vi "Untitled 1, Aula 4 (João).vi"() -> (1 "Potencia ativa A":dbl[](graph), 4 "Potencia ativa B":dbl[](graph), 7 "Potencia ativa C":dbl[](graph), 9 "timestamp":dbl[](array[numeric]))   [LabVIEW 2024]
uses:
  <vilib>/numeric/Random Number (Range) DBL.vi
panel:
  out "Tensão fase C":dbl[](array[numeric])
  out "Corrente fase C":dbl[](array[numeric])
  out "Potencia ativa":dbl[](array[numeric])
  out "Fator portencia 3":dbl
  in  "Limite inferior FP 3":dbl
  in  "Limite superior FP 3":dbl=100.0
  out "Corrente fase B":dbl[](array[numeric])
  out "Tensão fase B":dbl[](array[numeric])
  out "Potencia ativa B":dbl[](array[numeric])
  out "Fator portencia 2":dbl
  in  "Limite inferior FP 2":dbl
  in  "Limite superior FP 2":dbl=100.0
  out "Potencia ativa A":dbl[](array[numeric])
  out "Fator portencia":dbl
  out "Corrente fase A":dbl[](array[numeric])
  out "Tensão fase A":dbl[](array[numeric])
  in  "Limite inferior FP":dbl
  in  "Limite superior FP":dbl=100.0
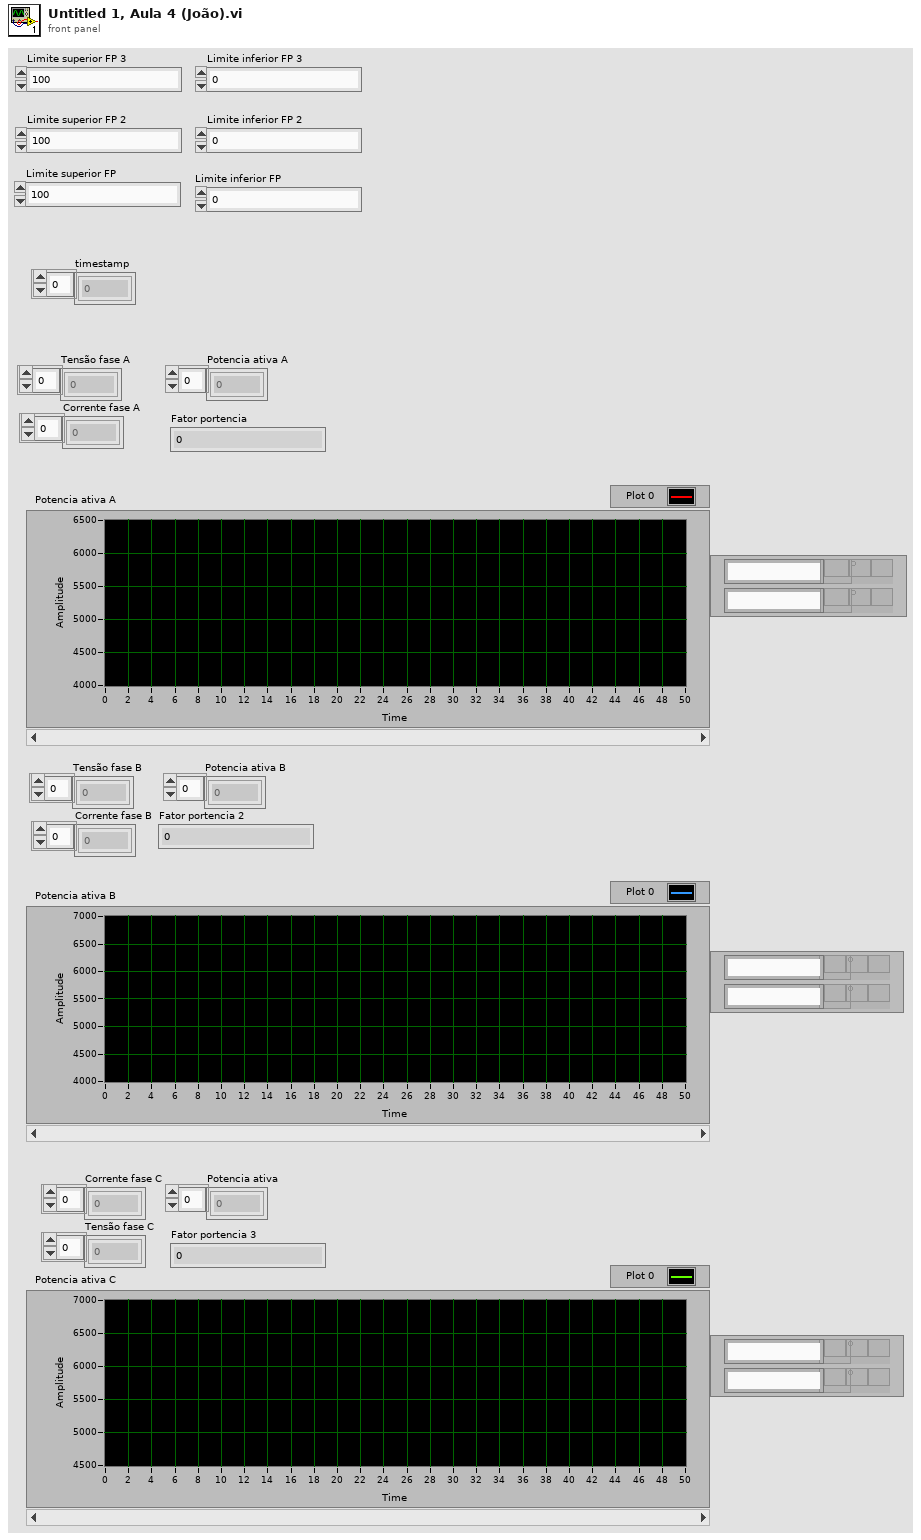
[diagram p1: front panel]
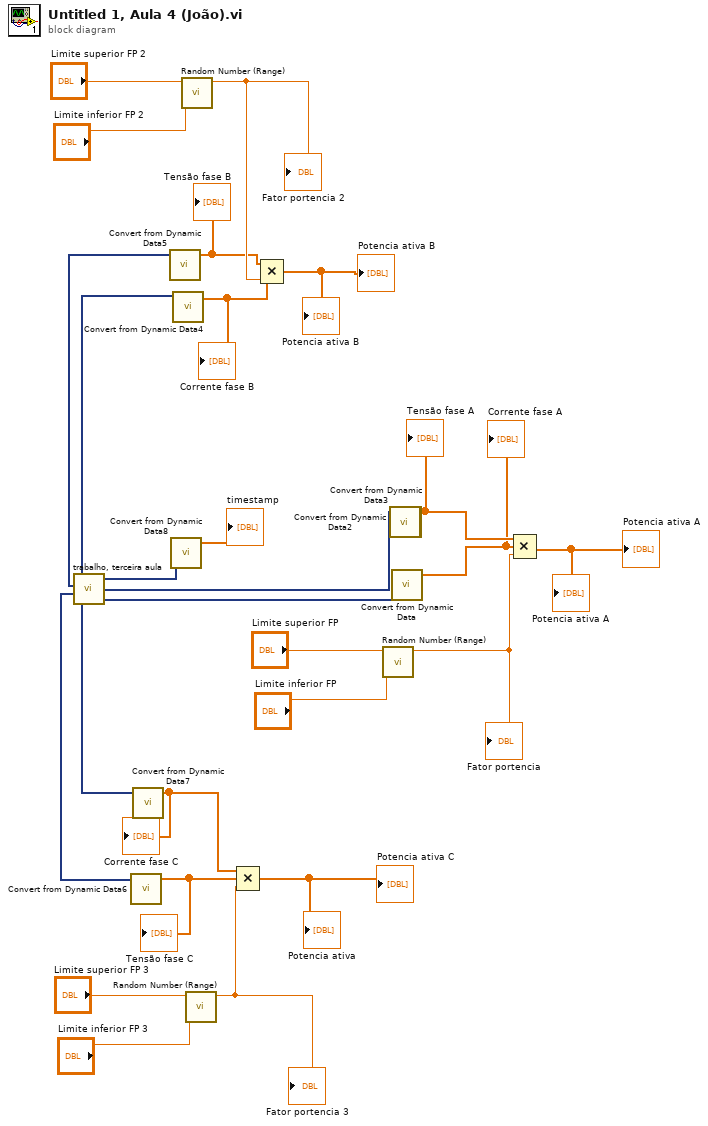
[diagram p0: block diagram]
diagram:
  n1 = call "trabalho, terceira aula.vi"() -> ("Corrente fase A"=w23:dynamicdata, "Tensão fase A"=w24:dynamicdata, "Timestamp"=w2:dynamicdata, "Corrente fase C"=w9:dynamicdata, "Tensão fase C"=w10:dynamicdata, "Corrente fase B"=w17:dynamicdata, "Tensão fase B"=w18:dynamicdata)
  n2 = call "Convert from Dynamic Data6"("Dynamic Data Type"=w10) -> ("Array"=w3:dbl[])  [unwired: 3 in]
  "Tensão fase C" <- w3
  n3 = call "Convert from Dynamic Data7"("Dynamic Data Type"=w9) -> ("Array"=w4:dbl[])  [unwired: 3 in]
  "Corrente fase C" <- w4
  n4 = call "Convert from Dynamic Data5"("Dynamic Data Type"=w17) -> ("Array"=w12:dbl[])  [unwired: 3 in]
  "Tensão fase B" <- w12
  n5 = call "Convert from Dynamic Data8"("Dynamic Data Type"=w2) -> ("Array"=→"timestamp":dbl[])  [unwired: 3 in]
  n6 = call "Convert from Dynamic Data4"("Dynamic Data Type"=w18) -> ("Array"=w11:dbl[])  [unwired: 3 in]
  "Corrente fase B" <- w11
  n7 = call-poly <vilib>:"Random Number (Range).vi"("lower bound (0)"="Limite inferior FP 2", "upper bound (100)"="Limite superior FP 2") -> ("number"=w14:dbl)  [unwired: 9 in]
  "Fator portencia 2" <- w14
  n8 = call-poly <vilib>:"Random Number (Range).vi"("lower bound (0)"="Limite inferior FP 3", "upper bound (100)"="Limite superior FP 3") -> ("number"=w6:dbl)  [unwired: 9 in]
  "Fator portencia 3" <- w6
  n9 = Compound Arithmetic op=MULTIPLY(w4, w3, w6) -> (→"Potencia ativa C" →"Potencia ativa":dbl[])
  n10 = Compound Arithmetic op=MULTIPLY(w12, w11, w14) -> (→"Potencia ativa B" →"Potencia ativa B":dbl[])
  n11 = call-poly <vilib>:"Random Number (Range).vi"("lower bound (0)"="Limite inferior FP", "upper bound (100)"="Limite superior FP") -> ("number"=w20:dbl)  [unwired: 9 in]
  "Fator portencia" <- w20
  n12 = call "Convert from Dynamic Data2"("Dynamic Data Type"=w24) -> ("Array"=w22:dbl[])  [unwired: 3 in]
  "Tensão fase A" <- w22
  n13 = call "Convert from Dynamic Data3"() -> ()  [unwired: 4 in, 1 out]
  n14 = call "Convert from Dynamic Data"("Dynamic Data Type"=w23) -> ("Array"=w21:dbl[])  [unwired: 3 in]
  "Corrente fase A" <- w21
  n15 = Compound Arithmetic op=MULTIPLY(w22, w21, w20) -> (→"Potencia ativa A" →"Potencia ativa A":dbl[])
